vi "Set Voltage Step.vi"(8 "error in (no error)":errorcluster, 10 "Voltage Step":string, 11 "Driver Test in":refnum<class "Driver Test.lvclass">) -> (0 "error out":errorcluster)   [LabVIEW 2015, in "Measurement.lvclass"]
uses:
  Measurement/Measurement.lvclass
  Driver Test.lvclass
  <vilib>/Cree, Inc/Cree Test Framework/Classes/Variable Engine/Class/Variable Engine.lvclass
  <vilib>/Cree, Inc/Cree Test Framework/Core Launcher/Core Launcher.lvlib
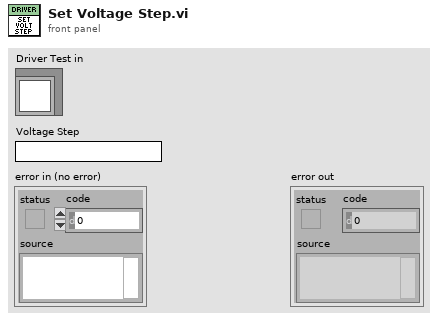
[diagram p1: front panel]
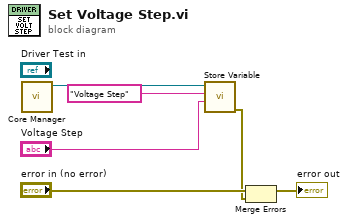
[diagram p0: block diagram]
diagram:
  n1 = call <vilib>:"Core Manager.vi"() -> ("Variable Engine"=w4:refnum<class "Variable Engine.lvclass">)  [unwired: 7 in, 4 out]
  n2 = call <vilib>:"Store Variable.vi"("Value"="Voltage Step", "Key"="Voltage Step", "Acrobat Template in"=w4) -> ("error out"=w1:errorcluster)  [unwired: 7 in, 1 out]
  n3 = Merge Errors("error in (no error)", w1) -> (→"error out":errorcluster)
